vi "opt_function_test2.vi"(9 "output selector":T1, 10 "data":variant, 11 "Initial parameters":dbl[](array[numeric])=[-0.257, 0.543, -0.0481, -0.0116]) -> (0 "error out":errorcluster, 1 "Inequality Constraints":dbl[](array[numeric]), 2 "Equality Constraints":dbl[](array[numeric]), 3 "Global Error":dbl[](array[numeric])=[4.856108225248919])   [LabVIEW 2020]
doc: "Finds the global minimum on a surface using the formula illustrated on the block diagram."
uses:
  <vilib>/gmath/NumericalOptimization/cno_output select.ctl
  Camera software flag.vi
  Global line error.vi
  <vilib>/gmath/NI_Gmath.lvlib
panel:
  out "Global line error 3":dbl=4.856108225248919
  out "Waveform Graph 2":dbl[](graph)
  out "Global line error 2":dbl
  out "Global line error":dbl=4.856108225248919
  in  "Save input parameter history":path=path "C:/Users/Hannah/Downloads/input parameters"
  in  "Save input parameters to file":bool
  in  "Flyback time (ms)":dbl=25.0
  in  "Acquisition time (ms)":dbl=100.0
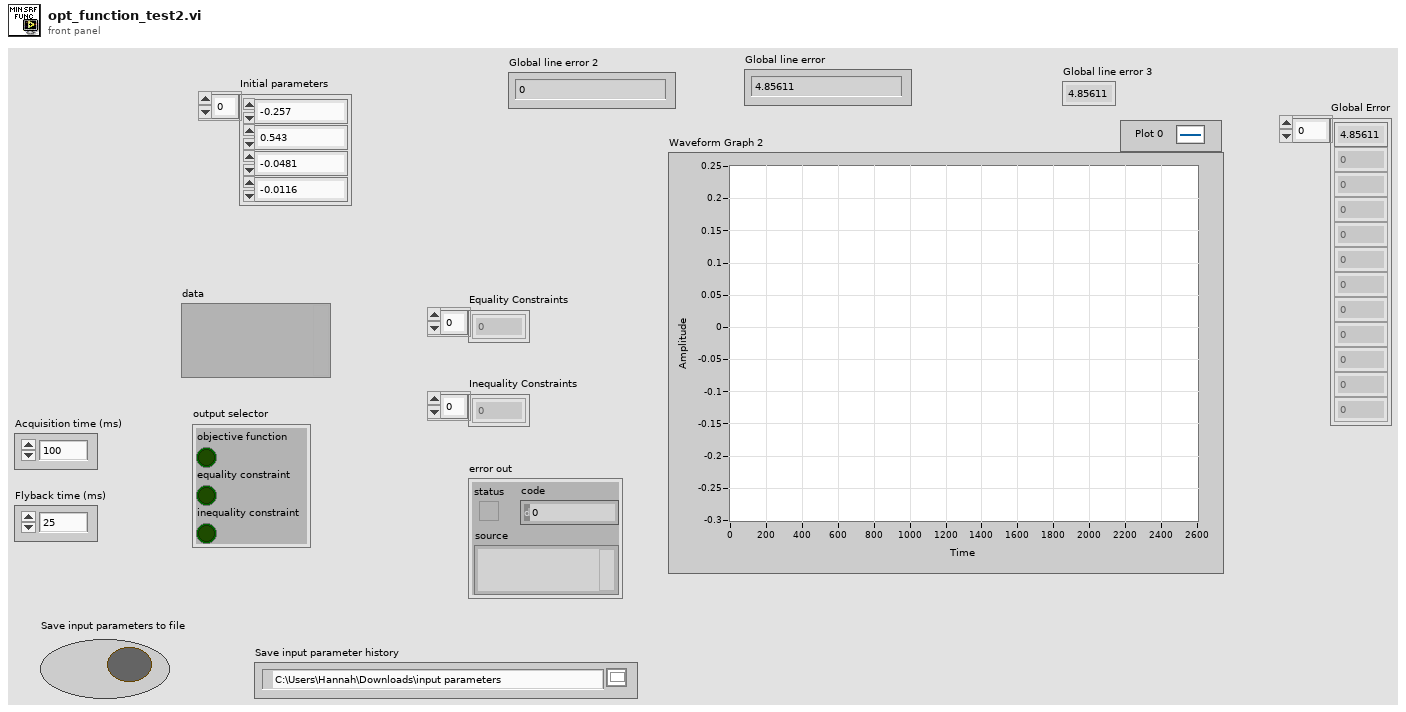
[diagram p1: front panel]
types:
  T1 = typedef "NI_Gmath.lvlib/cno_output select.ctl" = cluster{"objective function":bool, "equality constraint":bool, "inequality constraint":bool}
  T2 = enum16{"open", "replace", "create", "open or create", "replace or create", "replace or create with confirmation"}
  T3 = cluster{"Initial parameters[0]":dbl, "Initial parameters[1]":dbl, "Initial parameters[2]":dbl, "Initial parameters[3]":dbl, "Initial parameters[4]":dbl, "Initial parameters[5]":dbl, "Initial parameters[6]":dbl, "Initial parameters[7]":dbl, "Initial parameters[8]":dbl}
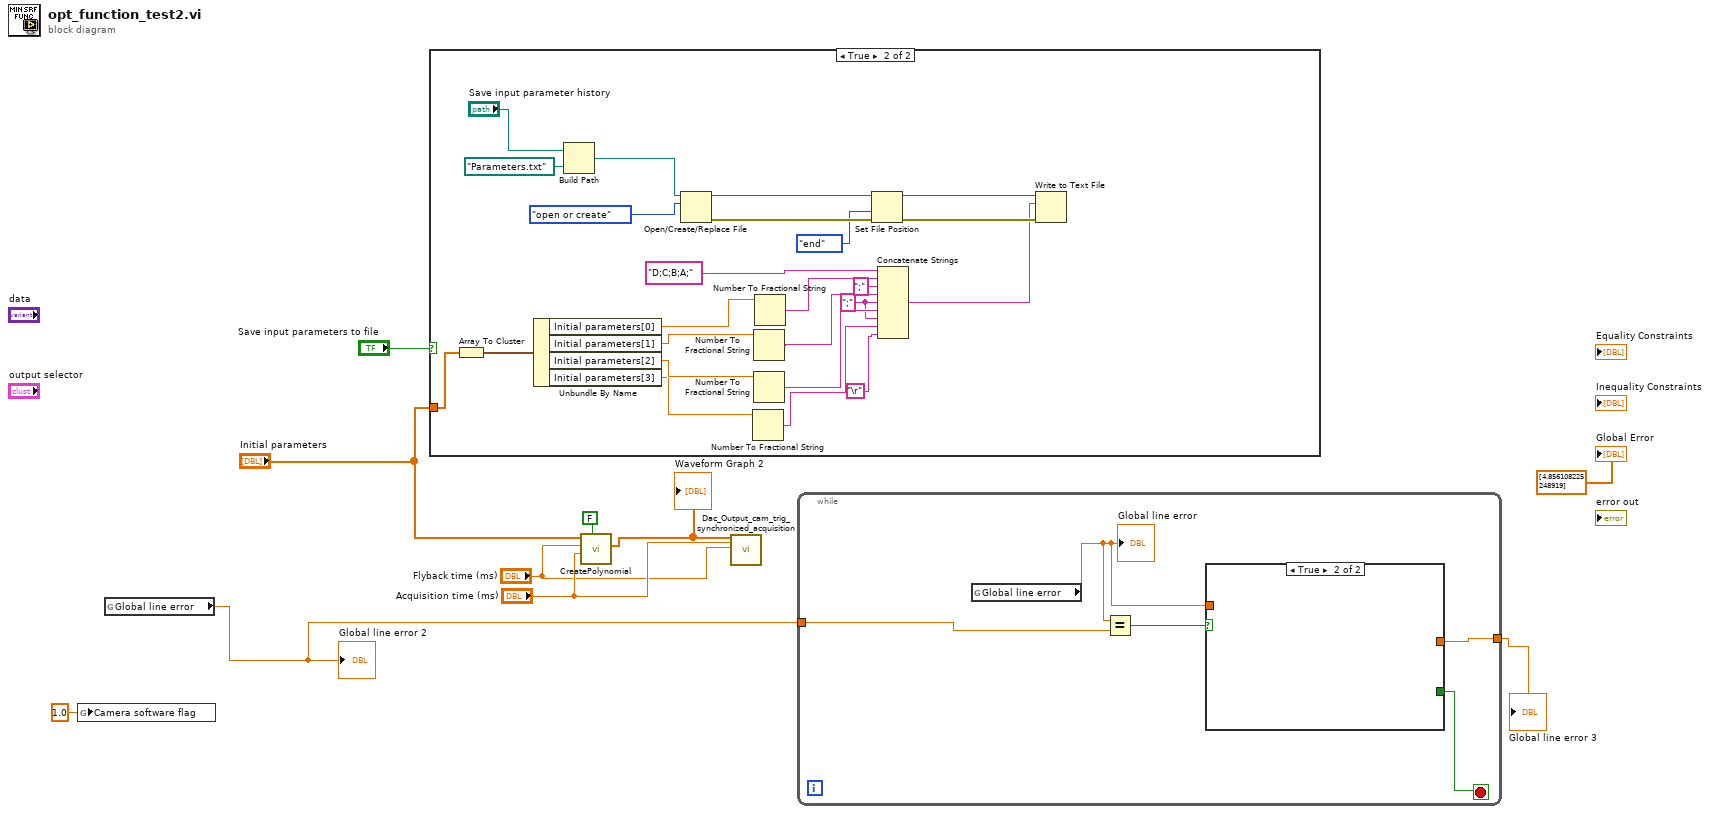
[diagram p0: block diagram]
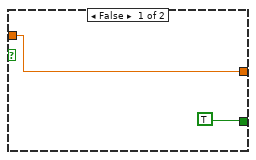
[diagram p2: hidden frame]
diagram:
  n1 = global write "Camera software flag.vi" "Camera software flag"(1.0 ("Camera software flag")) -> ()
  n2 = global read "Global line error.vi" "Global line error"() -> (w5:dbl)
  "Global line error 2" <- w5
  n3 = case shown="True" "Save input parameters to file" {
    tunnel: "Initial parameters" -> [_ w20]
    frame False {
    }
    frame True {
      w14 = ";" ("string")
      n4 = Array To Cluster(array=w20) -> (cluster=w19:T3)
      n5 = Unbundle By Name(w19) -> ("Initial parameters[0]"=w18:dbl, "Initial parameters[1]"=w17:dbl, "Initial parameters[2]"=w16:dbl, "Initial parameters[3]"=w13:dbl)
      n6 = Build Path(base path="Save input parameter history", name or relative path=path "Parameters.txt") -> (appended path=w34:path)
      n7 = Open/Create/Replace File(file path (use dialog)=w34, operation (0:open)=T2."open or create") -> (refnum out=w30:refnum<file>, error out=w31:errorcluster)  [unwired: 4 in, 1 out]
      n8 = Number To Fractional String(number=w13) -> (F-format string=w12:string)  [unwired: 3 in]
      n9 = Number To Fractional String(number=w17) -> (F-format string=w23:string)  [unwired: 3 in]
      n10 = Number To Fractional String(number=w16) -> (F-format string=w22:string)  [unwired: 3 in]
      n11 = Number To Fractional String(number=w18) -> (F-format string=w26:string)  [unwired: 3 in]
      n12 = Set File Position(refnum=w30, from (0:start)=enum16{"start", "end", "current"}."end", error in=w31) -> (refnum out=w32:refnum<file>, error out=w33:errorcluster)  [unwired: 1 in]
      n13 = Concatenate Strings("D;C;B;A;" ("text"), w26, ";" ("string"), w23, w14, w22, w14, w12, "\r") -> (w11:string)
      n14 = Write to Text File(file (use dialog)=w32, text=w11, error in=w33) -> ()  [unwired: 1 in, 3 out]
    }
  }
  n15 = call "CreatePolynomial.vi"("Save calibration"=FALSE, "Acquisition time (ms)"="Acquisition time (ms)", "Flyback (ms)"="Flyback time (ms)", "P(x)"="Initial parameters") -> ("Waveform Graph 2"=w6:dbl[])  [unwired: 5 in, 1 out]
  "Waveform Graph 2" <- w6
  n16 = call "Dac_Output_cam_trig_synchronized_acquisition.vi"("LabVIEW generated Sawtooth input"=w6, "Image acquisition time (ms)"="Acquisition time (ms)", "Delay between frames (ms)"="Flyback time (ms)") -> ()  [unwired: 17 in]
  n17 = while {
    tunnel: w5 -> [w39]
    tunnel: [w36] -> w2
    stop <- w35 stop-if-true
    n18 = global read "Global line error.vi" "Global line error"() -> (w37:dbl)
    "Global line error" <- w37
    n19 = Equal?(x=w37, y=w39) -> (x = y?=w38:bool)
    n20 = case shown="True" w38 {
      tunnel: w37 -> [w41 _]
      tunnel: [w41 _] -> w36
      tunnel: [TRUE _] -> w35
      frame False {
      }
      frame True {
      }
    }
  }
  "Global line error 3" <- w2
  "Global Error" <- dbl[] [4.856108225248919] ("Global Error")
